vi "Database connection example.vi"   [LabVIEW 2017]
uses:
  <vilib>/addons/database/Connection.llb/DB Tools Open Connec (Path).vi
  <vilib>/addons/database/Auxilliary.llb/DB Tools Format Datetime String (Time Stamp).vi
  <vilib>/addons/database/NI_Database_API.lvlib
types:
  T1 = typedef "NI_Database_API.lvlib/Conn ObjectReference.ctl" = refnum<k1>
  T2 = cluster{"date/time string":string, string, i64, i64, string}
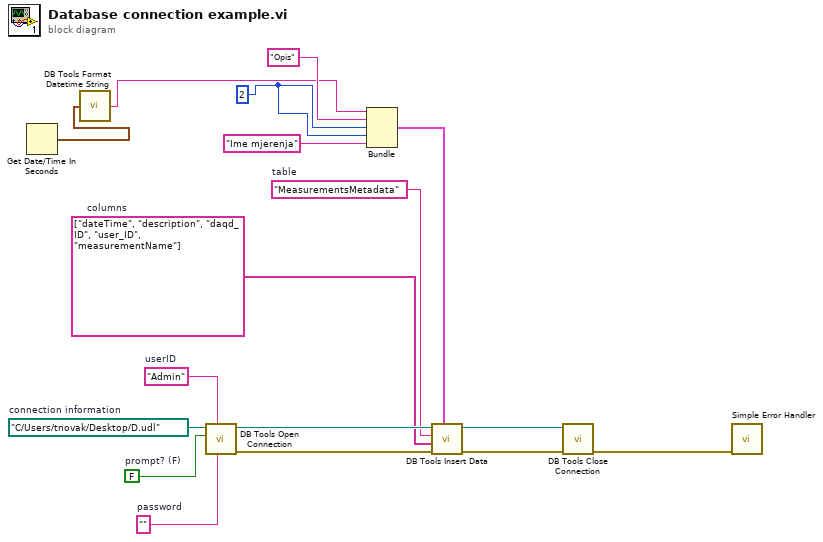
[diagram p0: block diagram]
diagram:
  w3 = i64 2
  w8 = "MeasurementsMetadata"  # table
  w7 = string[] ["dateTime", "description", "daqd_ID", "user_ID", "measurementName"]  # columns
  w13 = path "C:/Users/tnovak/Desktop/D.udl"  # connection information
  w15 = ""  # password
  w16 = FALSE  # prompt? (F)
  w17 = "Admin"  # userID
  n1 = Get Date/Time In Seconds() -> (seconds since 1Jan1904=w2:timestamp)
  n2 = call-poly <vilib>:"DB Tools Format Datetime String.vi"("time stamp"=w2) -> ("date/time string"=w1:string)
  n3 = call-poly <vilib>:"DB Tools Open Connection.vi"("password"=w15, "userID"=w17, "prompt? (F)"=w16, "connection information"=w13) -> ("error out"=w11:errorcluster, "connection reference"=w12:T1)  [unwired: 4 in]
  n4 = Bundle("date/time string"=w1, "Opis", w3, w3, "Ime mjerenja") -> (w4:T2)  [unwired: 1 in]
  n5 = call <vilib>:"DB Tools Insert Data.vi"("data"=w4, "error in (no error)"=w11, "columns"=w7, "table"=w8, "connection reference"=w12) -> ("error out"=w10:errorcluster, "connection reference out"=w9:T1)  [unwired: 5 in]
  n6 = call <vilib>:"DB Tools Close Connection.vi"("error in (no error)"=w10, "connection reference"=w9) -> ("error out"=w14:errorcluster)  [unwired: 5 in]
  n7 = call <vilib>:"Simple Error Handler.vi"("error in (no error)"=w14) -> ()  [unwired: 4 in, 5 out]
